vi "Temp Scene Update.vi"(5 "Property Name":T29, 6 "State":T31, 7 "Data Name":T30=enum."Property Class", 8 "error in (no error)":errorcluster, 11 "Property In":variant) -> (0 "error out":errorcluster, 3 "Multiplot Representation":T1)   [LabVIEW 2017, in "3D Plot.lvclass"]
uses:
  <vilib>/Math Plots/3D Math Plots/3D Plot/3D Plot/3D Plot.lvclass
  <vilib>/Math Plots/3D Math Plots/3D Plot/3D Plot/Typedef/Temp Scene State.ctl
  <vilib>/Math Plots/3D Math Plots/3D Plot/3D Plot/Typedef/Temp Scene Data Action.ctl
  <vilib>/Math Plots/3D Math Plots/3D Plot/3D Plot/Typedef/Temp Scene Property Action.ctl
  <vilib>/Math Plots/3D Math Plots/3D Plot/3D Plot/Typedef/Graph Property.ctl
  <vilib>/Math Plots/3D Math Plots/3D Plot/3D Plot/Typedef/General Property.ctl
  <vilib>/Math Plots/3D Math Plots/3D Plot/3D Plot/Typedef/View Property.ctl
  <vilib>/Math Plots/3D Math Plots/3D Plot/3D Plot/Typedef/Grid Plane.ctl
  <vilib>/Math Plots/3D Math Plots/3D Plot/3D Plot/Typedef/Light Property.ctl
  <vilib>/Math Plots/3D Math Plots/3D Plot/3D Plot/Typedef/Light Specific.ctl
  <vilib>/Math Plots/3D Math Plots/3D Plot/3D Plot/Typedef/Axis Property.ctl
  <vilib>/Math Plots/3D Math Plots/3D Plot/3D Plot/Typedef/Caption Property.ctl
  <vilib>/Math Plots/3D Math Plots/3D Plot/3D Plot/Typedef/Label Property.ctl
  <vilib>/Math Plots/3D Math Plots/3D Plot/3D Plot/Typedef/Range Property.ctl
  <vilib>/Math Plots/3D Math Plots/3D Plot/3D Plot/Typedef/Range Clusters.ctl
  <vilib>/Math Plots/3D Math Plots/3D Plot/3D Plot/Typedef/Grid Property.ctl
  <vilib>/Math Plots/3D Math Plots/3D Plot/3D Plot/Typedef/Tick Property.ctl
  <vilib>/Math Plots/3D Math Plots/3D Plot/3D Plot/Typedef/Value Pair Property.ctl
  <vilib>/Math Plots/3D Math Plots/3D Plot/3D Plot/Typedef/Value Pair Cluster.ctl
  <vilib>/Math Plots/3D Math Plots/3D Plot/3D Plot/Typedef/Format Property.ctl
  <vilib>/Math Plots/3D Math Plots/3D Plot/3D Plot/Typedef/Cursor Property Array.ctl
  <vilib>/Math Plots/3D Math Plots/3D Plot/3D Plot/Typedef/Cursor Property.ctl
  <vilib>/Math Plots/3D Math Plots/3D Plot/3D Plot/Typedef/Cursor Position.ctl
  <vilib>/Math Plots/3D Math Plots/3D Plot/3D Plot/Typedef/Cursor Point.ctl
  <vilib>/Math Plots/3D Math Plots/3D Plot/3D Plot/Typedef/Sprite Type.ctl
  <vilib>/Math Plots/3D Math Plots/3D Plot/3D Plot/Typedef/Cursor Line.ctl
  <vilib>/Math Plots/3D Math Plots/3D Plot/3D Plot/Typedef/Line Type.ctl
  <vilib>/Math Plots/3D Math Plots/3D Plot/3D Plot/Typedef/Cursor Plane.ctl
  <vilib>/Math Plots/3D Math Plots/3D Plot/3D Plot/Typedef/Cursor Text.ctl
  <vilib>/Math Plots/3D Math Plots/3D Plot/3D Plot/Typedef/Multiplot Representation.ctl
  <vilib>/Math Plots/3D Math Plots/3D Plot/3D Plot/Typedef/Plot Representation.ctl
  <vilib>/Math Plots/3D Math Plots/3D Plot/3D Plot/Typedef/Mesh Data.ctl
  <vilib>/Math Plots/3D Math Plots/3D Plot/3D Plot Datatype/3D Plot Datatype.lvclass
  <vilib>/Math Plots/3D Math Plots/3D Plot/3D Plot/Typedef/Object Cluster.ctl
  <vilib>/Math Plots/3D Math Plots/3D Plot/Action String/3DMathPlot Ctrl Act Queue.ctl
  <vilib>/Math Plots/3D Math Plots/3D Plot/Action String/3DMathPlot Ctrl Act Cluster.ctl
  <vilib>/Math Plots/3D Math Plots/3D Plot/Action String/3DMathPlot State Class.ctl
  <vilib>/Math Plots/3D Math Plots/3D Plot/3D Plot/3D Plot.lvclass/3D Plot.ctl
  <vilib>/Math Plots/3D Math Plots/3D Plot/3D Plot/Typedef/Actual Transform.ctl
panel:
  in  "Cursor Property Array":T5
  in  "Format Property":T14
  in  "Value Pair Property":T15
  in  "Axis Property":T17
  in  "Light Property":T23
  in  "Graph Property":T25
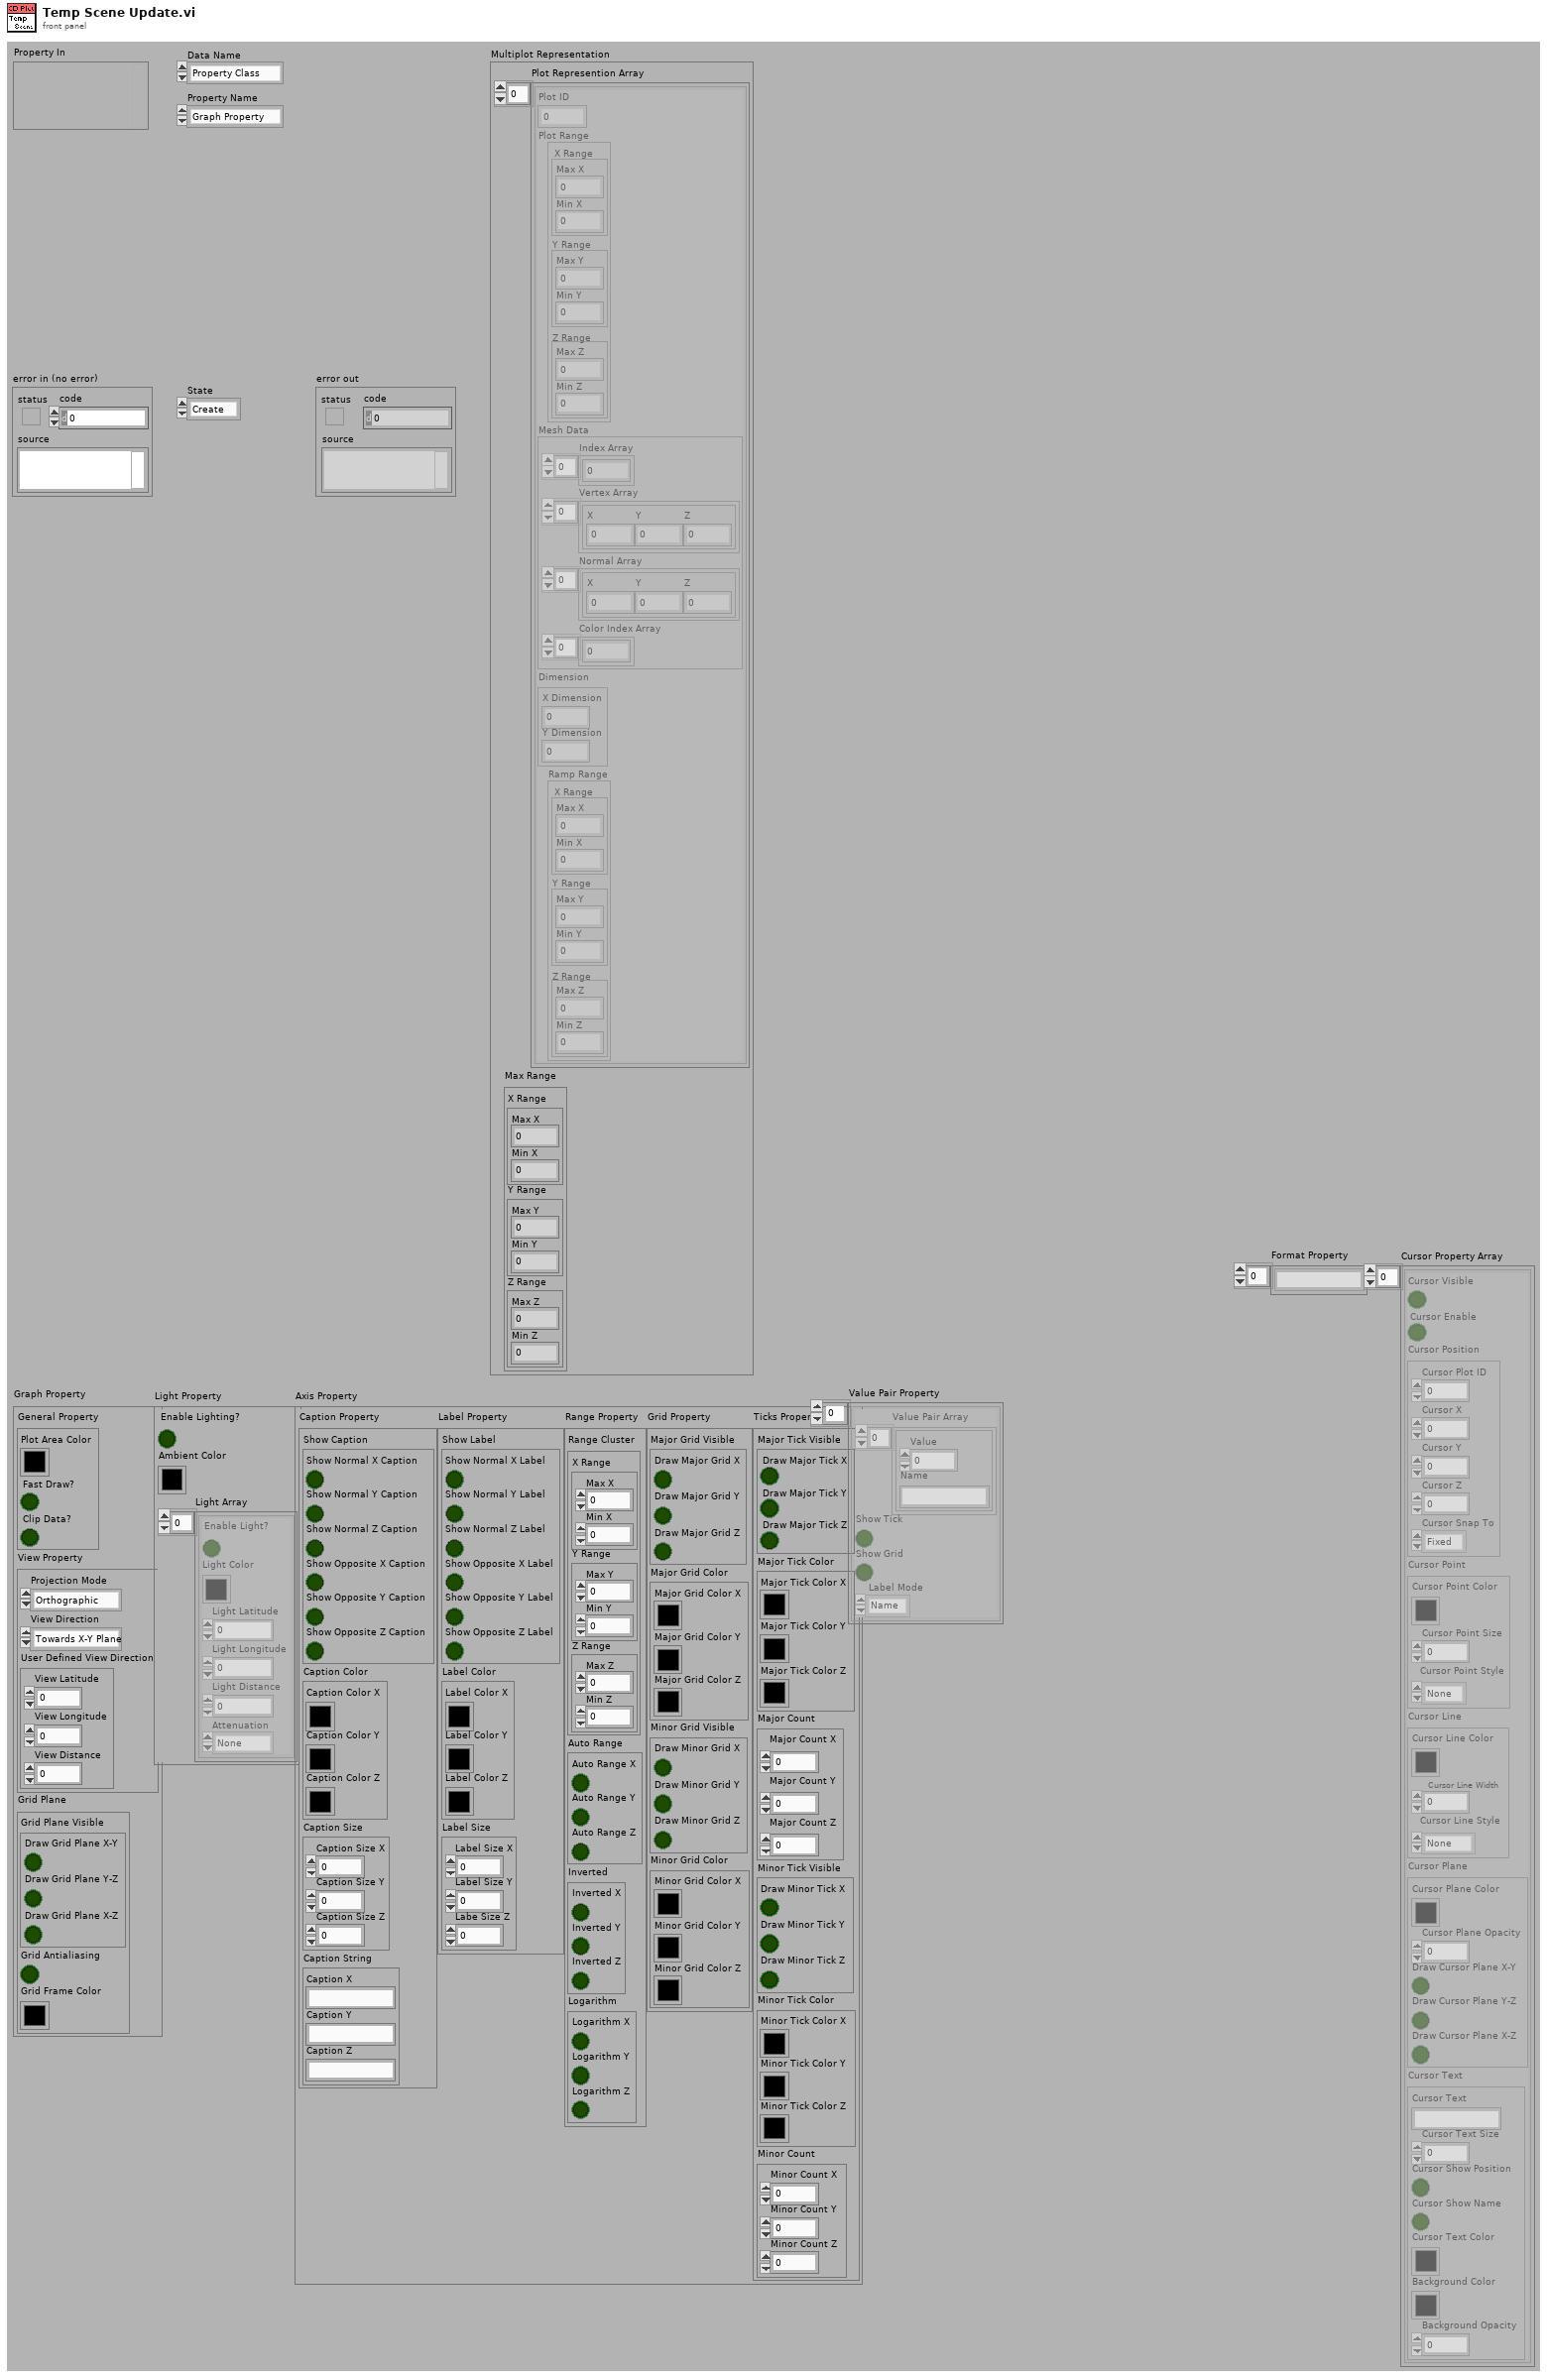
[diagram p1: front panel]
types:
  T1 = typedef "3D Plot.lvclass/Multiplot Representation.ctl" = cluster{"Plot Represention Array":T2[], "Max Range":T3}
  T2 = typedef "3D Plot.lvclass/Plot Representation.ctl" = cluster{"Plot ID":i32, "Plot Range":T3, "Mesh Data":T4, "Dimension":cluster{"X Dimension":i32, "Y Dimension":i32}, "Ramp Range":T3}
  T3 = typedef "3D Plot.lvclass/Range Clusters.ctl" = cluster{"X Range":cluster{"Max X":sgl, "Min X":sgl}, "Y Range":cluster{"Max Y":sgl, "Min Y":sgl}, "Z Range":cluster{"Max Z":sgl, "Min Z":sgl}}
  T4 = typedef "3D Plot.lvclass/Mesh Data.ctl" = cluster{"Index Array":u32[], "Vertex Array":cluster{"X":sgl, "Y":sgl, "Z":sgl}[], "Normal Array":cluster{"X":sgl, "Y":sgl, "Z":sgl}[], "Color Index Array":i32[]}
  T5 = typedef "3D Plot.lvclass/Cursor Property Array.ctl" = T6[]
  T6 = typedef "3D Plot.lvclass/Cursor Property.ctl" = cluster{"Cursor Visible":bool, "Cursor Enable":bool, "Cursor Position":T7, "Cursor Point":T8, "Cursor Line":T10, "Cursor Plane":T12, "Cursor Text":T13}
  T7 = typedef "3D Plot.lvclass/Cursor Position.ctl" = cluster{"Cursor Plot ID":i32, "Cursor X":sgl, "Cursor Y":sgl, "Cursor Z":sgl, "Cursor Snap To":enum16{"Fixed", "Nearest Plot", "Snap to Plot"}}
  T8 = typedef "3D Plot.lvclass/Cursor Point.ctl" = cluster{"Cursor Point Color":u32, "Cursor Point Size":sgl, "Cursor Point Style":T9}
  T9 = typedef "3D Plot.lvclass/Sprite Type.ctl" = enum16{"None", "Empty Square", "Solid Square", "Empty Diamond", "Solid Diamond", "Empty Circle", "Solid Circle", "Asterisk", "Bold X", "Wireframe Sphere", "Solid Sphere", "Wireframe Cube", "Solid Cube"}
  T10 = typedef "3D Plot.lvclass/Cursor Line.ctl" = cluster{"Cursor Line Color":u32, "Cursor Line Width":sgl, "Cursor Line Style":T11}
  T11 = typedef "3D Plot.lvclass/Line Type.ctl" = enum16{"None", "Solid", "Dash", "Dot", "Dash Dot"}
  T12 = typedef "3D Plot.lvclass/Cursor Plane.ctl" = cluster{"Cursor Plane Color":u32, "Cursor Plane Opacity":sgl, "Draw Cursor Plane X-Z":bool, "Draw Cursor Plane Y-Z":bool, "Draw Cursor Plane X-Y":bool}
  T13 = typedef "3D Plot.lvclass/Cursor Text.ctl" = cluster{"Cursor Text":string, "Cursor Text Size":u16, "Cursor Show Position":bool, "Cursor Show Name":bool, "Cursor Text Color":u32, "Background Color":u32, "Background Opacity":sgl}
  T14 = typedef "3D Plot.lvclass/Format Property.ctl" = string[]
  T15 = typedef "3D Plot.lvclass/Value Pair Property.ctl" = T16[]
  T16 = typedef "3D Plot.lvclass/Value Pair Cluster.ctl" = cluster{"Value Pair Array":cluster{"Value":sgl, "Name":string}[], "Show Tick":bool, "Show Grid":bool, " Label Mode":enum16{"Name", "Value", "None"}}
  T17 = typedef "3D Plot.lvclass/Axis Property.ctl" = cluster{"Caption Property":T18, "Label Property":T19, "Range Property":T20, "Grid Property":T21, "Ticks Property":T22}
  T18 = typedef "3D Plot.lvclass/Caption Property.ctl" = cluster{"Show Caption":cluster{"Show Normal X Caption":bool, "Show Normal Y Caption":bool, "Show Normal Z Caption":bool, "Show Opposite X Caption":bool, "Show Opposite Y Caption":bool, "Show Opposite Z Caption":bool}, "Caption Color":cluster{"Caption Color X":u32, "Caption Color Y":u32, "Caption Color Z":u32}, "Caption Size":cluster{"Caption Size X":u16, "Caption Size Y":u16, "Caption Size Z":u16}, "Caption String":cluster{"Caption X":string, "Caption Y":string, "Caption Z ":string}}
  T19 = typedef "3D Plot.lvclass/Label Property.ctl" = cluster{"Show Label":cluster{"Show Normal X Label":bool, "Show Normal Y Label":bool, "Show Normal Z Label":bool, "Show Opposite X Label":bool, "Show Opposite Y Label":bool, "Show Opposite Z Label":bool}, "Label Color":cluster{"Label Color X":u32, "Label Color Y":u32, "Label Color Z":u32}, "Label Size":cluster{"Label Size X":u16, "Label Size Y":u16, "Labe Size Z":u16}}
  T20 = typedef "3D Plot.lvclass/Range Property.ctl" = cluster{"Range Cluster":T3, "Auto Range":cluster{"Auto Range X":bool, "Auto Range Y":bool, "Auto Range Z":bool}, "Inverted":cluster{"Inverted X":bool, "Inverted Y":bool, "Inverted Z":bool}, "Logarithm":cluster{"Logarithm X":bool, "Logarithm Y":bool, "Logarithm Z":bool}}
  T21 = typedef "3D Plot.lvclass/Grid Property.ctl" = cluster{"Major Grid Visible":cluster{"Draw Major Grid X":bool, "Draw Major Grid Y":bool, "Draw Major Grid Z":bool}, "Major Grid Color":cluster{"Major Grid Color X":u32, "Major Grid Color Y":u32, "Major Grid Color Z":u32}, "Minor Grid Visible":cluster{"Draw Minor Grid X":bool, "Draw Minor Grid Y":bool, "Draw Minor Grid Z":bool}, "Minor Grid Color":cluster{"Minor Grid Color X":u32, "Minor Grid Color Y":u32, "Minor Grid Color Z":u32}}
  T22 = typedef "3D Plot.lvclass/Tick Property.ctl" = cluster{"Major Tick Visible":cluster{"Draw Major Tick X":bool, "Draw Major Tick Y":bool, "Draw Major Tick Z":bool}, "Major Tick Color":cluster{"Major Tick Color X":u32, "Major Tick Color Y":u32, "Major Tick Color Z":u32}, "Major Count":cluster{"Major Count X":u16, "Major Count Y":u16, "Major Count Z":u16}, "Minor Tick Visible":cluster{"Draw Minor Tick X":bool, "Draw Minor Tick Y":bool, "Draw Minor Tick Z":bool}, "Minor Tick Color":cluster{"Minor Tick Color X":u32, "Minor Tick Color Y":u32, "Minor Tick Color Z":u32}, "Minor Count":cluster{"Minor Count X":u16, "Minor Count Y":u16, "Minor Count Z":u16}}
  T23 = typedef "3D Plot.lvclass/Light Property.ctl" = cluster{"Enable Lighting?":bool, "Ambient Color":u32, "Light Array":T24[]}
  T24 = typedef "3D Plot.lvclass/Light Specific.ctl" = cluster{"Enable Light?":bool, "Light Color":u32, "Light Latitude":sgl, "Light Longitude":sgl, "Light Distance":sgl, "Attenuation":enum16{"None", "Linear", "Quadratic"}}
  T25 = typedef "3D Plot.lvclass/Graph Property.ctl" = cluster{"General Property":T26, "View Property":T27, "Grid Plane":T28}
  T26 = typedef "3D Plot.lvclass/General Property.ctl" = cluster{"Plot Area Color":u32, "Fast Draw?":bool, "Clip Data?":bool}
  T27 = typedef "3D Plot.lvclass/View Property.ctl" = cluster{"Projection Mode":enum16{"Orthographic", "Perspective"}, "View Direction":enum32{"Towards X-Y Plane", "Towards X-Z Plane", "Towards Y-Z Plane", "User Defined"}, "User Defined View Direction":cluster{"View Latitude":sgl, "View Longitude":sgl, "View Distance":sgl}}
  T28 = typedef "3D Plot.lvclass/Grid Plane.ctl" = cluster{"Grid Plane Visible":cluster{"Draw Grid Plane X-Y":bool, "Draw Grid Plane Y-Z":bool, "Draw Grid Plane X-Z":bool}, "Grid Antialiasing":bool, "Grid Frame Color":u32}
  T29 = typedef "3D Plot.lvclass/Temp Scene Property Action.ctl" = enum16{"Graph Property", "Light Property", "Axis Property", "Value Pair Property", "Format Property", "Cursor Property", "Plot Specific Property"}
  T30 = typedef "3D Plot.lvclass/Temp Scene Data Action.ctl" = enum16{"Data Class", "Property Class", "Object Cluster", "Control Queue"}
  T31 = typedef "3D Plot.lvclass/Temp Scene State.ctl" = enum16{"Create", "Update Scene", "Get Plot Representation", "Destory"}
  T32 = typedef "3D Plot.lvclass/Object Cluster.ctl" = cluster{"Root Scene Object":refnum<vi>, "Fast Root Scene Object":refnum<vi>}
  T33 = typedef "3DMathPlot Ctrl Act Queue.ctl" = refnum<queue>
  T34 = typedef "3DMathPlot State Class.ctl" = enum16{"Update All Objects (Undo)", "Update Light Object Only", "Update Axis Object Only", "Update Plot Object Only", "Update Cursor Object Only", "Update Axis Plot Cursor Objects", "No Update"}
  T35 = typedef "3D Plot.lvclass/Actual Transform.ctl" = cluster{"Scale Cluster":cluster{"X Scale":sgl, "Y Scale":sgl, "Z Scale":sgl}, "Translate Cluster":cluster{"X Translate":sgl, "Y Translate":sgl, "Z Translate":sgl}, "Actual Range":T3}
  T36 = enum32{"Towards X-Y Plane", "Towards X-Z Plane", "Towards Y-Z Plane", "User Defined"}
  T37 = typedef "3D Plot.lvclass/Plot Action.ctl" = cluster{"Light Action":enum16{"Update", "Remove", "Nothing"}, "Axis Action":enum16{"Update", "Remove", "Nothing"}, "Plot Action":enum16{"Update", "Remove", "Nothing"}, "Cursor Action":enum16{"Update", "Remove", "Nothing"}, "Fast Draw Action":enum16{"Update", "Remove", "Nothing"}}
  T38 = typedef "3DMathPlot Ctrl Act Cluster.ctl" = cluster{"3D Picture Control":refnum<vi>, "Render Window Refnum":refnum<vi>, "XY Graph":refnum<vi>, "Intensity Graph":refnum<vi>, "Color Legend Palette":refnum<vi>, "Projection Palette":refnum<vi>, "XControl  Ref":refnum<vi>, "Facade Ref":refnum<vi>, "Export Image Ref":refnum<vi>, "Clear Data Flag":bool, "Display State Change Class":T34}
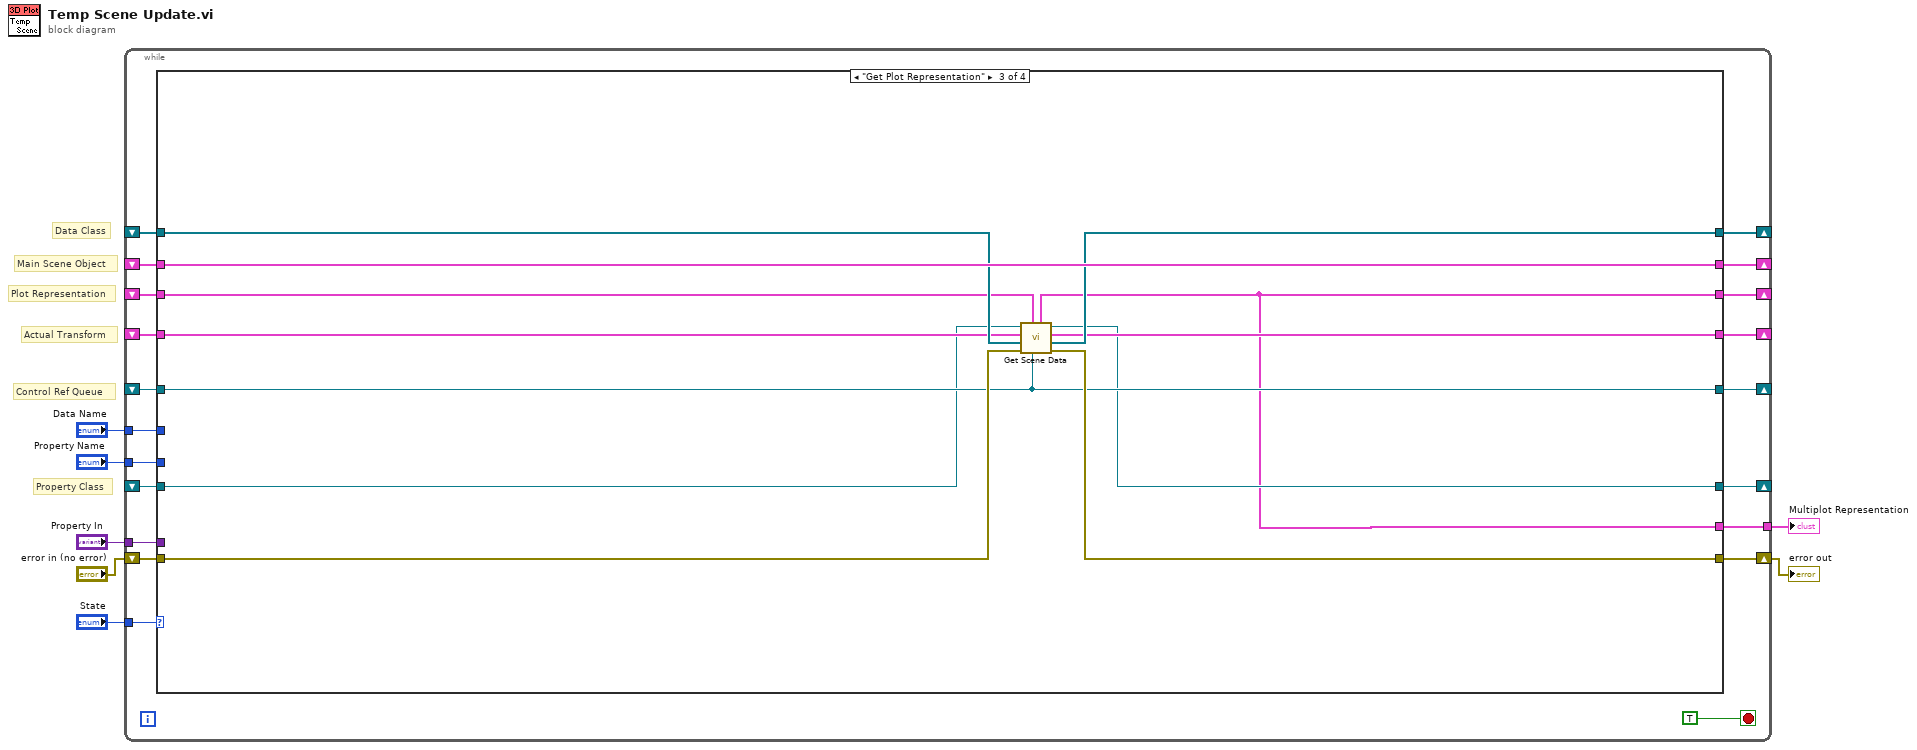
[diagram p0: block diagram]
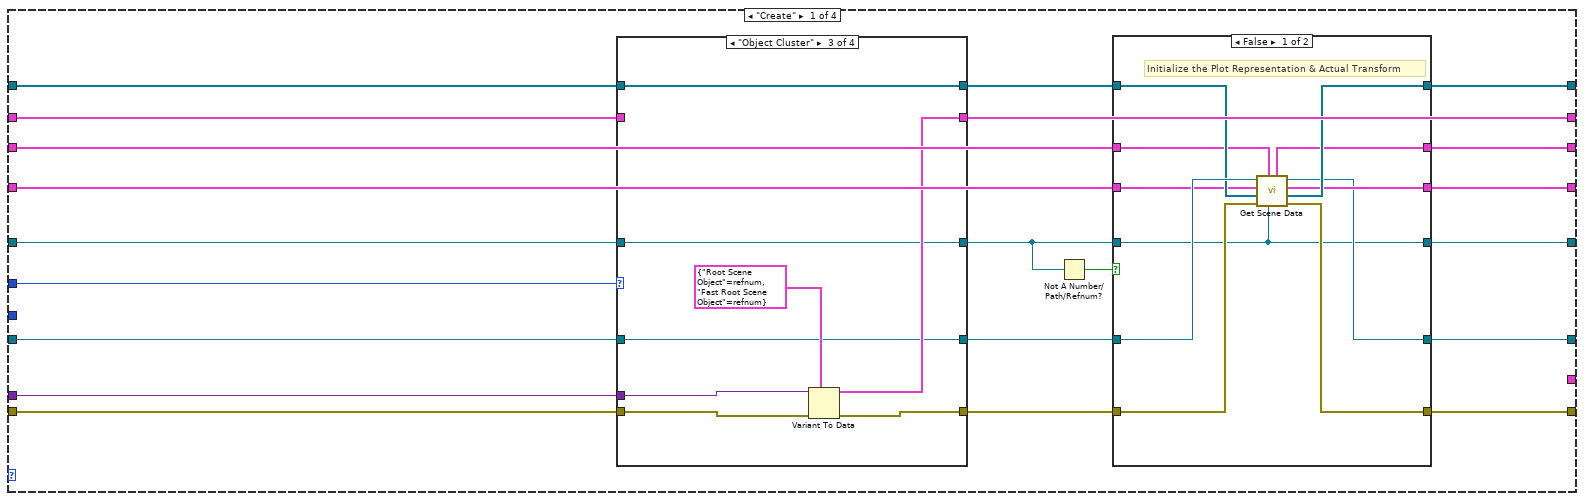
[diagram p2: hidden frame]
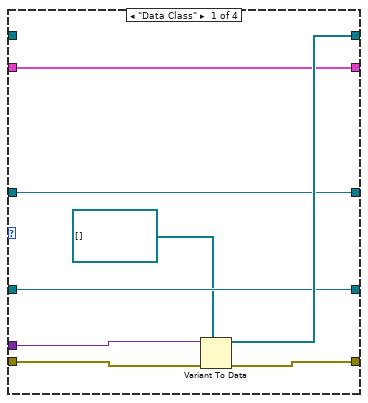
[diagram p4: hidden frame]
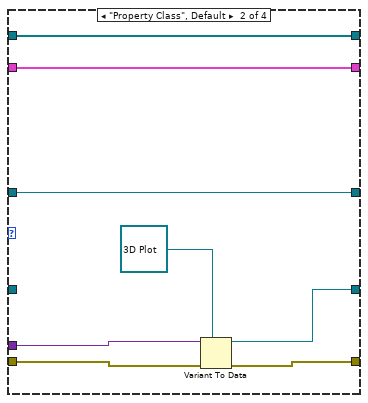
[diagram p5: hidden frame]
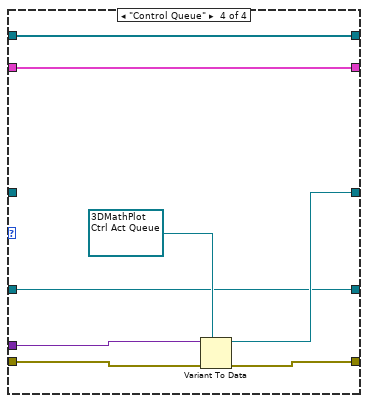
[diagram p6: hidden frame]
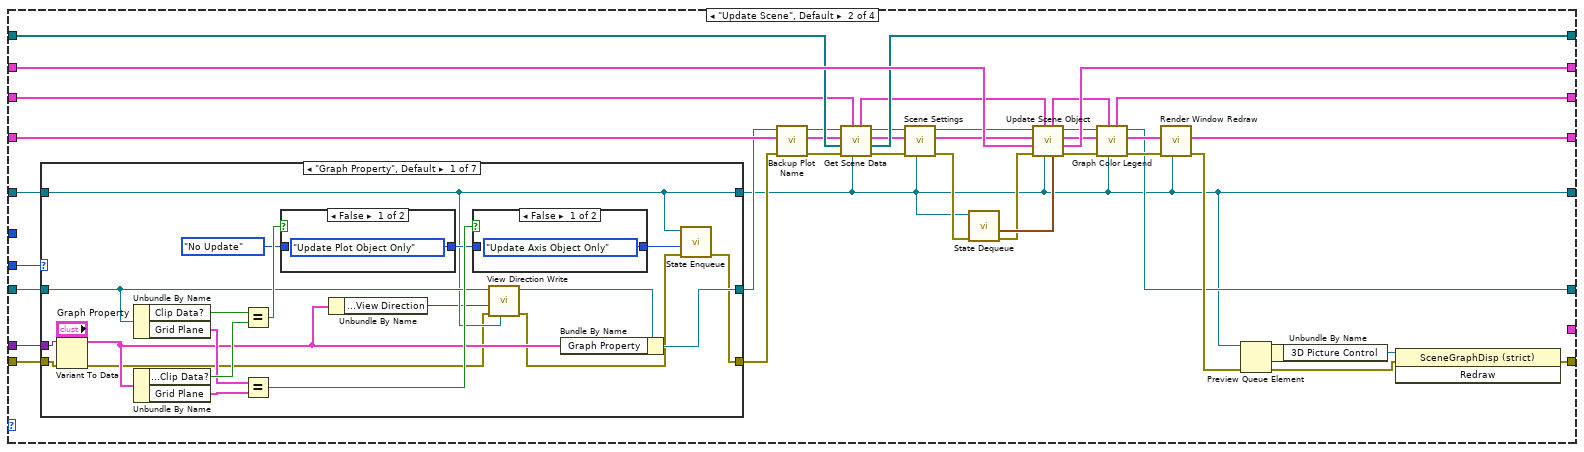
[diagram p7: hidden frame]
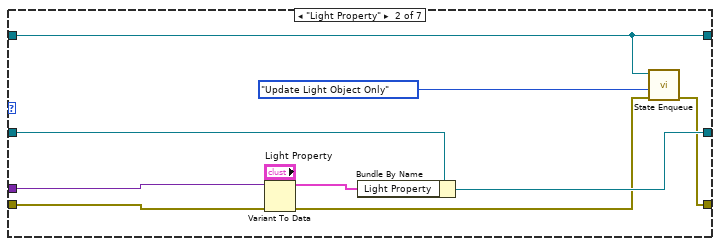
[diagram p10: hidden frame]
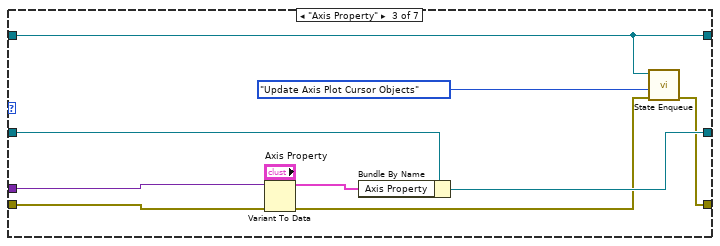
[diagram p11: hidden frame]
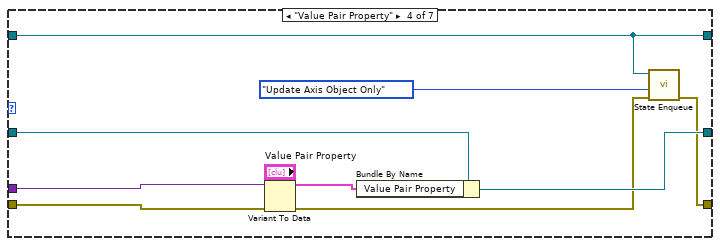
[diagram p12: hidden frame]
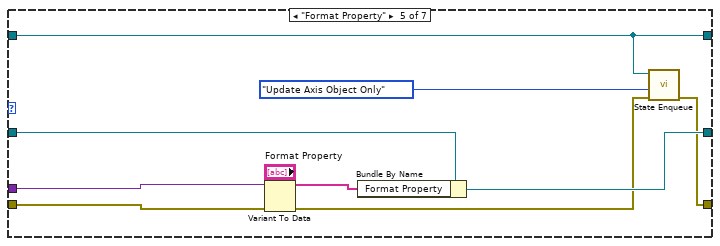
[diagram p13: hidden frame]
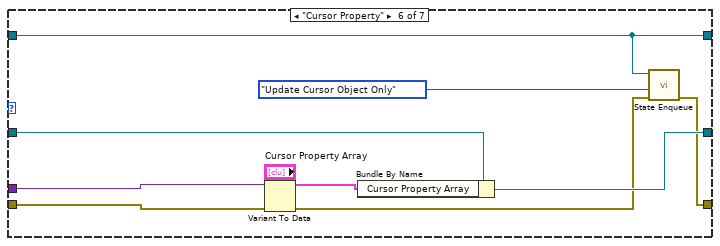
[diagram p14: hidden frame]
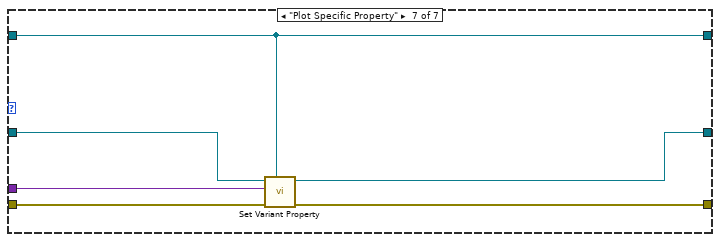
[diagram p15: hidden frame]
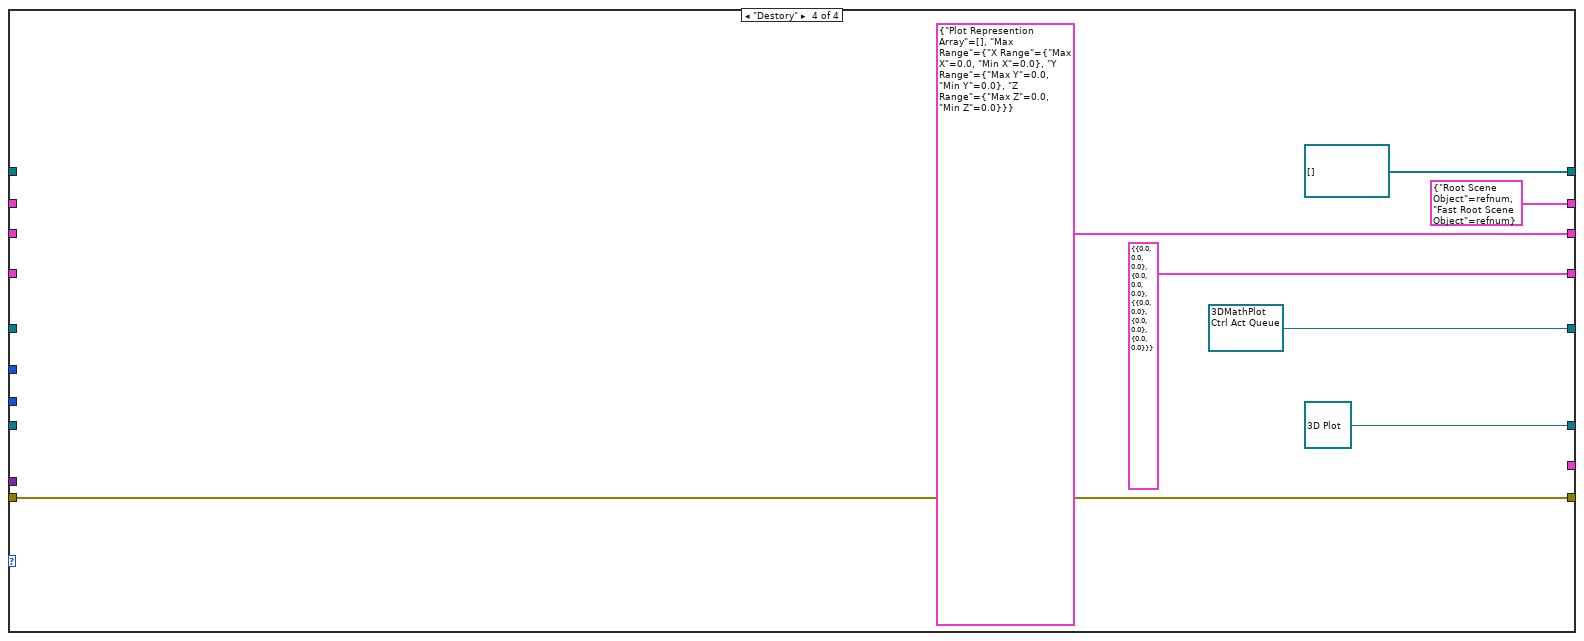
[diagram p16: hidden frame]
diagram:
  # "Plot Representation"
  # "Actual Transform"
  # "Control Ref Queue"
  # "Main Scene Object"
  # "Data Class"
  # "Property Class"
  n1 = while {
    tunnel: "State" -> [w26]
    tunnel: "Property In" -> [w25]
    tunnel: "Data Name" -> [w24]
    shift-right: [w23] -> _
    shift-left: _ -> [w20]
    shift-right: [w21] -> w2
    shift-left: "error in (no error)" -> [w22]
    shift-right: [w19] -> _
    shift-left: _ -> [w18]
    shift-right: [w17] -> _
    shift-left: _ -> [w15]
    shift-right: [w16] -> _
    shift-left: _ -> [w14]
    tunnel: "Property Name" -> [w13]
    shift-right: [w12] -> _
    shift-left: _ -> [w11]
    tunnel: [w10] -> w1
    shift-right: [w9] -> _
    shift-left: _ -> [w8]
    stop <- TRUE stop-if-true
    n2 = case shown="\"Get Plot Representation\"" w26 {
      tunnel: w25 -> [w47 w133 _ _]
      tunnel: w24 -> [w48 _ _ _]
      tunnel: [w33 w103 w217 refnum<class "3D Plot.lvclass"> refnum ("3D Plot.lvclass in")] -> w23
      tunnel: w22 -> [w46 w132 w226 w233]
      tunnel: [w31 w126 w225 w233] -> w21
      tunnel: w20 -> [w45 w104 w218 _]
      tunnel: [w38 w123 w222 refnum<class "3D Plot Datatype.lvclass">[] []] -> w19
      tunnel: w18 -> [w44 w124 w223 _]
      tunnel: [w43 w130 w227 T32 {"Root Scene Object"=refnum, "Fast Root Scene Object"=refnum} ("Object Cluster Out")] -> w17
      tunnel: [w28 w98 w224 T33 refnum ("Control Ref Queue")] -> w16
      tunnel: w15 -> [w42 w131 w227 _]
      tunnel: w14 -> [w41 w99 w224 _]
      tunnel: w13 -> [_ w134 _ _]
      tunnel: [w36 w120 w216 T1 {"Plot Represention Array"=[], "Max Range"={"X Range"={"Max X"=0.0, "Min X"=0.0}, "Y Range"={"Max Y"=0.0, "Min Y"=0.0}, "Z Range"={"Max Z"=0.0, "Min Z"=0.0}}} ("Multiplot Representation Out")] -> w12
      tunnel: w11 -> [w37 w121 w221 _]
      tunnel: [_ _ w216 _] -> w10
      tunnel: [w34 w119 w219 T35 {"Scale Cluster"={"X Scale"=0.0, "Y Scale"=0.0, "Z Scale"=0.0}, "Translate Cluster"={"X Translate"=0.0, "Y Translate"=0.0, "Z Translate"=0.0}, "Actual Range"={"X Range"={"Max X"=0.0, "Min X"=0.0}, "Y Range"={"Max Y"=0.0, "Min Y"=0.0}, "Z Range"={"Max Z"=0.0, "Min Z"=0.0}}} ("Actual Transform Out")] -> w9
      tunnel: w8 -> [w35 w122 w220 _]
      frame "Create" {
        n3 = case shown="\"Object Cluster\"" w48 {
          tunnel: w47 -> [w71 w81 w88 w96]
          tunnel: [w69 w74 w82 w92] -> w40
          tunnel: w46 -> [w73 w79 w85 w94]
          tunnel: [w72 w78 w86 w93] -> w32
          tunnel: [w70 w77 w83 w91] -> w39
          tunnel: w45 -> [w69 _ w82 w92]
          tunnel: w44 -> [_ w77 w83 w91]
          tunnel: [w68 w76 w87 w90] -> w43
          tunnel: [w67 w75 w84 w95] -> w30
          tunnel: w42 -> [w68 w76 _ w90]
          tunnel: w41 -> [w67 w75 w84 _]
          frame "Data Class" {
            n4 = Variant To Data(error in=w73, type=refnum<class "3D Plot Datatype.lvclass">[] [], Variant=w71) -> (data=w70:refnum<class "3D Plot Datatype.lvclass">[], error out=w72:errorcluster)
          }
          frame "Property Class", Default {
            n5 = Variant To Data(error in=w79, type=refnum<class "3D Plot.lvclass"> refnum ("3D Plot.lvclass in"), Variant=w81) -> (data=w74:refnum<class "3D Plot.lvclass">, error out=w78:errorcluster)
          }
          frame "Object Cluster" {
            n6 = Variant To Data(error in=w85, type=T32 {"Root Scene Object"=refnum, "Fast Root Scene Object"=refnum} ("Object Cluster Out"), Variant=w88) -> (data=w87:T32, error out=w86:errorcluster)
          }
          frame "Control Queue" {
            n7 = Variant To Data(error in=w94, type=T33 refnum ("Control Ref Queue"), Variant=w96) -> (data=w95:T33, error out=w93:errorcluster)
          }
        }
        n8 = Not A Number/Path/Refnum?(number/path/refnum=w30) -> (NaN/Path/Refnum?=w29:bool)
        n9 = case shown="False" w29 {
          tunnel: w40 -> [w59 w62]
          tunnel: w39 -> [w58 w65]
          tunnel: [w57 w65] -> w38
          tunnel: w37 -> [w56 w64]
          tunnel: [w55 w64] -> w36
          tunnel: w35 -> [w54 w63]
          tunnel: [w53 w63] -> w34
          tunnel: w30 -> [w49 w60]
          tunnel: [w52 w62] -> w33
          tunnel: w32 -> [w51 w61]
          tunnel: [w50 w61] -> w31
          tunnel: [w49 w60] -> w28
          frame False {
            # "Initialize the Plot Representation & Actual Transform"
            n10 = call <vilib>:"Get Scene Data.vi"("Control Ref Queue"=w49, "Multiplot Representation In"=w56, "error in (no error)"=w51, "Data In"=w58, "Actual Transform In"=w54, "3D Plot.lvclass in"=w59) -> ("error out"=w50:errorcluster, "Data Out"=w57:refnum<class "3D Plot Datatype.lvclass">[], "Actual Transform Out"=w53:T35, "3D Plot.lvclass out"=w52:refnum<class "3D Plot.lvclass">, "Multiplot Representation Out"=w55:T1)  [unwired: 1 out]
          }
          frame True {
          }
        }
      }
      frame "Update Scene", Default {
        n11 = case shown="\"Graph Property\", Default" w134 {
          tunnel: w133 -> [w154 w166 w175 w189 w199 w209 w212]
          tunnel: w132 -> [w153 w165 w174 w184 w195 w204 w215]
          tunnel: w104 -> [w141 w168 w176 w187 w198 w206 w214]
          tunnel: [w155 w164 w177 w185 w194 w205 w213] -> w118
          tunnel: [w151 w160 w171 w182 w191 w201 w211] -> w116
          tunnel: w99 -> [w139 w162 w170 w180 w192 w203 w210]
          tunnel: [w139 w162 w170 w180 w192 w203 w210] -> w98
          frame "Graph Property", Default {
            n12 = Variant To Data(error in=w153, type="Graph Property", Variant=w154) -> (data=w138:T25, error out=w136:errorcluster)
            n13 = Unbundle By Name(w141) -> ("Clip Data?"=w150:bool, "Grid Plane"=w147:T28)
            n14 = Unbundle By Name(w138) -> ("General Property.Clip Data?"=w149:bool, "Grid Plane"=w146:T28)
            n15 = Equal?(x=w150, y=w149) -> (x = y?=w148:bool)
            n16 = Equal?(x=w147, y=w146) -> (x = y?=w145:bool)
            n17 = case shown="False" w148 {
              tunnel: [3DMathPlot_State_Class."Update Plot Object Only" ("Display State Change Class") w159] -> w143
              tunnel: 3DMathPlot_State_Class."No Update" ("Display State Change Class") -> [_ w159]
              frame False {
              }
              frame True {
              }
            }
            n18 = Unbundle By Name(w138) -> ("View Property.View Direction"=w137:T36)
            n19 = case shown="False" w145 {
              tunnel: [3DMathPlot_State_Class."Update Axis Object Only" ("Display State Change Class") w157] -> w144
              tunnel: w143 -> [_ w157]
              frame False {
              }
              frame True {
              }
            }
            n20 = call <vilib>:"View Direction Write.vi"("Control Ref Queue"=w139, "error in (no error)"=w136, "View Direction"=w137, "3D Plot.lvclass in"=w141) -> ("error out"=w135:errorcluster, "3D Plot.lvclass out"=w140:refnum<class "3D Plot.lvclass">)  [unwired: 6 out]
            n21 = Bundle By Name(cluster=w140, "Graph Property"=w138) -> (w155:refnum<class "3D Plot.lvclass">)
            n22 = call <vilib>:"State Enqueue.vi"("error in (no error)"=w135, "Display State Change Class"=w144, "Control Ref Queue"=w139) -> ("error out"=w151:errorcluster)  [unwired: 8 out]
          }
          frame "Light Property" {
            n23 = Variant To Data(error in=w165, type="Light Property", Variant=w166) -> (data=w167:T23, error out=w161:errorcluster)
            n24 = Bundle By Name(cluster=w168, "Light Property"=w167) -> (w164:refnum<class "3D Plot.lvclass">)
            n25 = call <vilib>:"State Enqueue.vi"("error in (no error)"=w161, "Display State Change Class"=3DMathPlot_State_Class."Update Light Object Only", "Control Ref Queue"=w162) -> ("error out"=w160:errorcluster)  [unwired: 8 out]
          }
          frame "Axis Property" {
            n26 = Variant To Data(error in=w174, type="Axis Property", Variant=w175) -> (data=w178:T17, error out=w172:errorcluster)
            n27 = Bundle By Name(cluster=w176, "Axis Property"=w178) -> (w177:refnum<class "3D Plot.lvclass">)
            n28 = call <vilib>:"State Enqueue.vi"("error in (no error)"=w172, "Display State Change Class"=3DMathPlot_State_Class."Update Axis Plot Cursor Objects", "Control Ref Queue"=w170) -> ("error out"=w171:errorcluster)  [unwired: 8 out]
          }
          frame "Value Pair Property" {
            n29 = Variant To Data(error in=w184, type="Value Pair Property", Variant=w189) -> (data=w186:T15, error out=w181:errorcluster)
            n30 = Bundle By Name(cluster=w187, "Value Pair Property"=w186) -> (w185:refnum<class "3D Plot.lvclass">)
            n31 = call <vilib>:"State Enqueue.vi"("error in (no error)"=w181, "Display State Change Class"=3DMathPlot_State_Class."Update Axis Object Only", "Control Ref Queue"=w180) -> ("error out"=w182:errorcluster)  [unwired: 8 out]
          }
          frame "Format Property" {
            n32 = Variant To Data(error in=w195, type="Format Property", Variant=w199) -> (data=w197:T14, error out=w190:errorcluster)
            n33 = Bundle By Name(cluster=w198, "Format Property"=w197) -> (w194:refnum<class "3D Plot.lvclass">)
            n34 = call <vilib>:"State Enqueue.vi"("error in (no error)"=w190, "Display State Change Class"=3DMathPlot_State_Class."Update Axis Object Only", "Control Ref Queue"=w192) -> ("error out"=w191:errorcluster)  [unwired: 8 out]
          }
          frame "Cursor Property" {
            n35 = Variant To Data(error in=w204, type="Cursor Property Array", Variant=w209) -> (data=w207:T5, error out=w202:errorcluster)
            n36 = Bundle By Name(cluster=w206, "Cursor Property Array"=w207) -> (w205:refnum<class "3D Plot.lvclass">)
            n37 = call <vilib>:"State Enqueue.vi"("error in (no error)"=w202, "Display State Change Class"=3DMathPlot_State_Class."Update Cursor Object Only", "Control Ref Queue"=w203) -> ("error out"=w201:errorcluster)  [unwired: 8 out]
          }
          frame "Plot Specific Property" {
            n38 = call-dynamic "Set Variant Property.vi"("Control Ref Queue"=w210, "error in (no error)"=w215, "Property In"=w212, "3D Plot.lvclass in"=w214) -> ("error out"=w211:errorcluster, "3D Plot.lvclass"=w213:refnum<class "3D Plot.lvclass">)  [unwired: 1 in, 5 out]
          }
        }
        n39 = call-dynamic "Backup Plot Name.vi"("error in (no error)"=w116, "3D Plot.lvclass in"=w118) -> ("error out"=w108:errorcluster, "3D Plot.lvclass out"=w111:refnum<class "3D Plot.lvclass">)  [unwired: 8 out]
        n40 = call <vilib>:"Get Scene Data.vi"("Control Ref Queue"=w98, "Multiplot Representation In"=w121, "error in (no error)"=w108, "Data In"=w124, "Actual Transform In"=w122, "3D Plot.lvclass in"=w111) -> ("error out"=w109:errorcluster, "Data Out"=w123:refnum<class "3D Plot Datatype.lvclass">[], "Actual Transform Out"=w107:T35, "3D Plot.lvclass out"=w110:refnum<class "3D Plot.lvclass">, "Multiplot Representation Out"=w106:T1)  [unwired: 1 out]
        n41 = call <vilib>:"Scene Settings.vi"("Control Ref Queue"=w98, "error in (no error)"=w109, "Actual Transform In"=w107, "3D Plot.lvclass in"=w110) -> ("error out"=w101:errorcluster, "Actual Transform Out"=w114:T35, "3D Plot.lvclass out"=w112:refnum<class "3D Plot.lvclass">)  [unwired: 3 in, 2 out]
        n42 = call <vilib>:"State Dequeue.vi"("error in (no error)"=w101, "Control Ref Queue"=w98) -> ("error out"=w100:errorcluster, "Action"=w102:T37)  [unwired: 8 out]
        n43 = call <vilib>:"Update Scene Object.vi"("Action"=w102, "Control Ref Queue"=w98, "Multiplot Representation In"=w106, "error in (no error)"=w100, "Object Cluster In"=w131, "Actual Transform In"=w114, "3D Plot.lvclass in"=w112) -> ("error out"=w115:errorcluster, "Object Cluster Out"=w130:T32, "Actual Transform Out"=w119:T35, "3D Plot.lvclass out"=w117:refnum<class "3D Plot.lvclass">, "Multiplot Representation Out"=w105:T1)
        n44 = call-dynamic "Graph Color Legend.vi"("Control Ref Queue"=w98, "Multiplot Representation In"=w105, "error in (no error)"=w115, "3D Plot.lvclass in"=w117) -> ("error out"=w113:errorcluster, "3D Plot.lvclass out"=w103:refnum<class "3D Plot.lvclass">, "Multiplot Representation Out"=w120:T1)  [unwired: 2 in, 3 out]
        n45 = call <vilib>:"Render Window Redraw.vi"("Control Ref Queue"=w98, "error in (no error)"=w113) -> ("error out"=w125:errorcluster)  [unwired: 9 out]
        n46 = Preview Queue Element(queue=w98, error in (no error)=w125) -> (element=w129:T38, error out=w127:errorcluster)  [unwired: 3 out]
        n47 = Unbundle By Name(w129) -> ("3D Picture Control"=w128:refnum<vi>)
        n48 = invoke class="SceneGraphDisp (strict)" method="Redraw"(reference=w128, error in=w127) -> (error out=w126:errorcluster)  [unwired: 1 in, 2 out]
      }
      frame "Get Plot Representation" {
        n49 = call <vilib>:"Get Scene Data.vi"("Control Ref Queue"=w224, "Multiplot Representation In"=w221, "error in (no error)"=w226, "Data In"=w223, "Actual Transform In"=w220, "3D Plot.lvclass in"=w218) -> ("error out"=w225:errorcluster, "Data Out"=w222:refnum<class "3D Plot Datatype.lvclass">[], "Actual Transform Out"=w219:T35, "3D Plot.lvclass out"=w217:refnum<class "3D Plot.lvclass">, "Multiplot Representation Out"=w216:T1)  [unwired: 1 out]
      }
      frame "Destory" {
      }
    }
  }
  "error out" <- w2
  "Multiplot Representation" <- w1
